vi "Examine Configuration.vi"(8 "error in (no error)":errorcluster, 11 "Instrument in":refnum<class "Instrument.lvclass">) -> (0 "error out":errorcluster, 3 "Instrument out":refnum<class "Instrument.lvclass">)   [LabVIEW 2019, in "Instrument.lvlib" / "Instrument.lvclass"]
uses:
  Instrument.lvclass
  <userlib>/LevyLab/Configuration/Configuration.lvclass
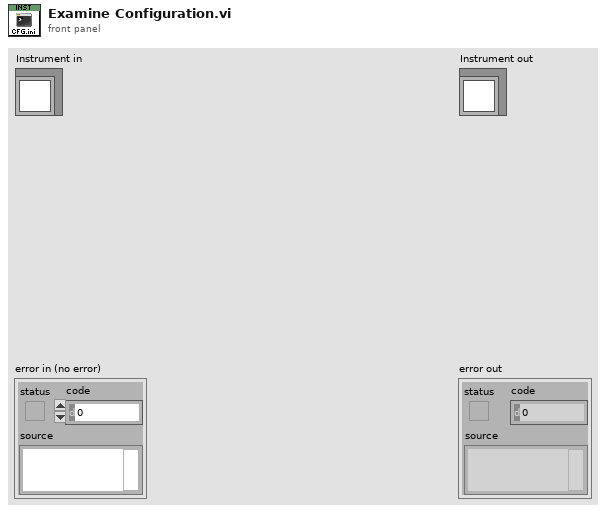
[diagram p1: front panel]
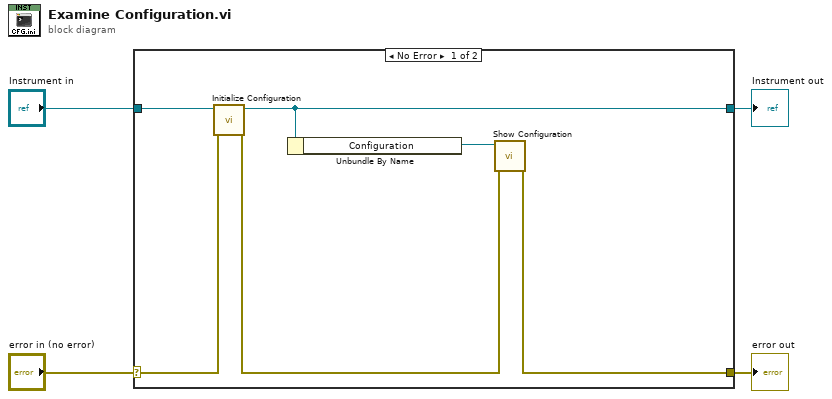
[diagram p0: block diagram]
diagram:
  n1 = case shown="No Error" "error in (no error)" {
    selector: "error in (no error)" -> [w6 w12]
    tunnel: [w9 w12] -> w3
    tunnel: [w8 w11] -> w1
    tunnel: "Instrument in" -> [w7 w11]
    frame No Error {
      n2 = call "Initialize Configuration.vi"("error in (no error)"=w6, "Instrument in"=w7) -> ("error out"=w5:errorcluster, "Instrument out"=w8:refnum<class "Instrument.lvclass">)  [unwired: 8 in]
      n3 = Unbundle By Name(w8) -> ("Configuration"=w10:refnum<class "Configuration.lvclass">)
      n4 = call <userlib>:"Show Configuration.vi"("error in (no error)"=w5, "Configuration in"=w10) -> ("error out"=w9:errorcluster)  [unwired: 8 in, 1 out]
    }
    frame Error {
    }
  }
  "error out" <- w3
  "Instrument out" <- w1
